vi "ListItems.vi"(8 "error in (no error)":errorcluster, 10 "Listbox":refnum<vi>, 11 "ObserverFactory in":refnum<class "ObserverFactory.lvclass">) -> (0 "error out":errorcluster, 3 "ObserverFactory out":refnum<class "ObserverFactory.lvclass">)   [LabVIEW 2020, in "ObserverFactory.lvclass"]
uses:
  ObserverFactory.lvclass
  ObserverFactory.lvclass/ObserverFactory.ctl
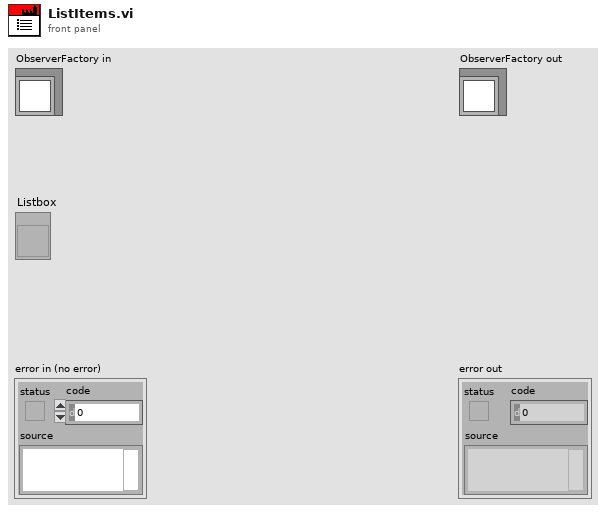
[diagram p1: front panel]
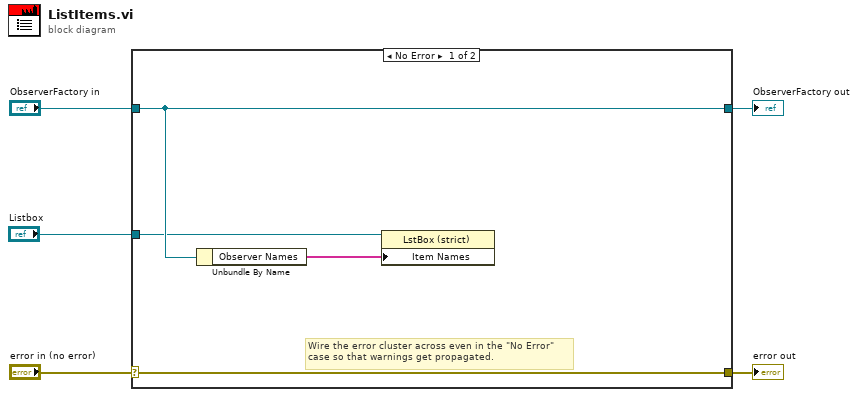
[diagram p0: block diagram]
diagram:
  n1 = case shown="No Error" "error in (no error)" {
    selector: "error in (no error)" -> [w9 w11]
    tunnel: [w9 w11] -> w4
    tunnel: [w8 w10] -> w2
    tunnel: "ObserverFactory in" -> [w8 w10]
    tunnel: "Listbox" -> [w7 _]
    frame No Error {
      # "Wire the error cluster across even in the \"No Error\"\ncase so that warnings get propagated."
      n2 = Unbundle By Name(w8) -> ("Observer Names"=w6:string[])
      n3 = property class="LstBox (strict)"(reference=w7, "Item Names"=w6) -> ()  [unwired: 1 in, 2 out]
    }
    frame Error {
    }
  }
  "error out" <- w4
  "ObserverFactory out" <- w2
